vi "UART_Str_Open.vi"(8 "error in":errorcluster, 9 "parity (0:none)":enum16{"None", "Odd", "Even", "Mark", "Space"}(ring), 10 "baud rate (115200)":u32=115200, 11 "VISA resource name":refnum<visa-resource-name>="COM1") -> (0 "error out":errorcluster, 3 "VISA resource name out":refnum<visa-resource-name>="COM1")   [LabVIEW 2015, in "UARTCOM.lvlib"]
uses:
  UARTCOM.lvlib
  <vilib>/Instr/_visa.llb/VISA Configure Serial Port (Instr).vi
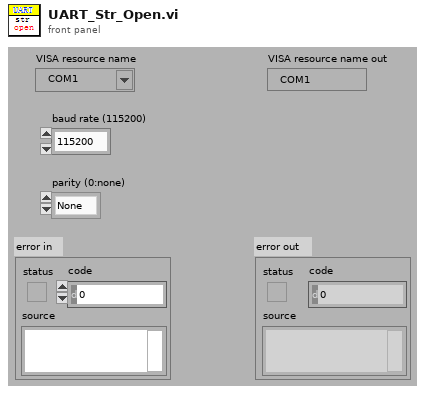
[diagram p1: front panel]
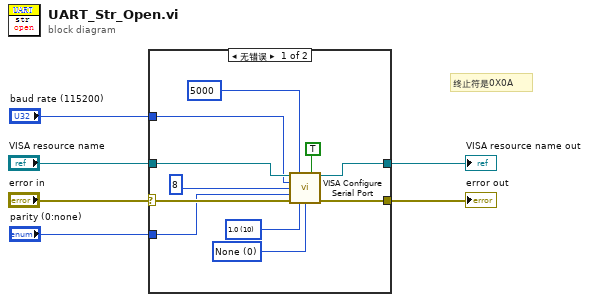
[diagram p0: block diagram]
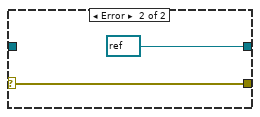
[diagram p2: hidden frame]
diagram:
  # "终止符是0X0A"
  n1 = case shown="无错误" "error in" {
    selector: "error in" -> [w15 w19]
    tunnel: [w17 w19] -> w5
    tunnel: [w16 refnum<visa-resource-name> refnum ("VISA resource name out")] -> w3
    tunnel: "VISA resource name" -> [w14 _]
    tunnel: "baud rate (115200)" -> [w10 _]
    tunnel: "parity (0:none)" -> [w9 _]
    frame No Error {
      w11 = u16 0 items=["None", "XON/XOFF", "RTS/CTS", "XON/XOFF & RTS/CTS", "DTR/DSR", "XON/XOFF & DTR/DSR"] ("flow control (0:none)")
      w12 = u16 10 items=["1.0"=10, "1.5"=15, "2.0"=20] ("stop bits (10: 1 bit)")
      n2 = call-poly "VISA Configure Serial Port"("VISA resource name"=w14, "timeout (10sec)"=u32 5000, "Enable Termination\nChar (T)"=TRUE ("Enable Termination\nChar (T)"), "baud rate (9600)"=w10, "data bits (8)"=u16 8, "parity (0:none)"=w9, "error in (no error)"=w15, "stop bits (10: 1 bit)"=w12, "flow control (0:none)"=w11) -> ("VISA resource name out"=w16:refnum<visa-resource-name>, "error out"=w17:errorcluster)  [unwired: 5 in]
    }
    frame Error {
    }
  }
  "error out" <- w5
  "VISA resource name out" <- w3
